vi "Find API Tester Path.vi"(8 "error in":errorcluster, 11 "DQMH Library Ref":refnum<vi>) -> (0 "error out":errorcluster, 3 "API Tester Path":path)   [LabVIEW 2020, in "Dashboard.lvlib"]
uses:
  Dashboard.lvlib
  <vilib>/Utility/error.llb/Error Cluster From Error Code.vi
  <vilib>/ErrorRing/Error Ring.xnode
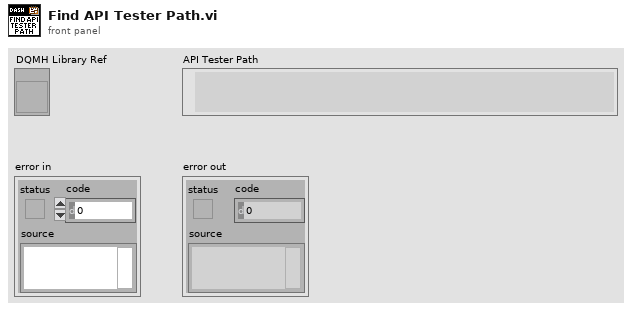
[diagram p1: front panel]
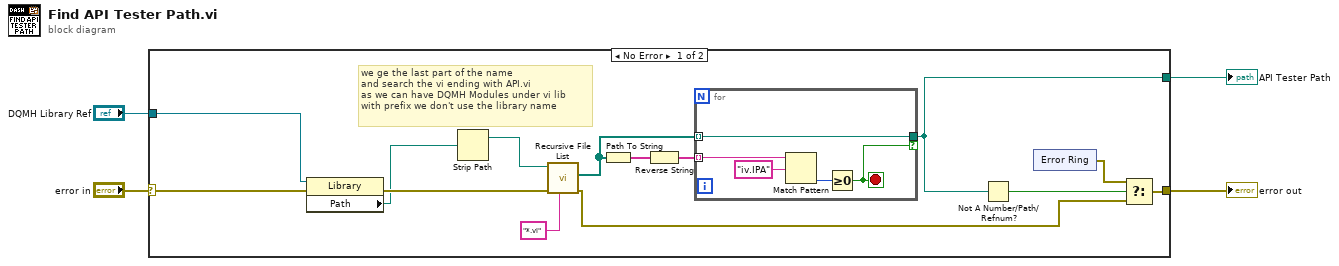
[diagram p0: block diagram]
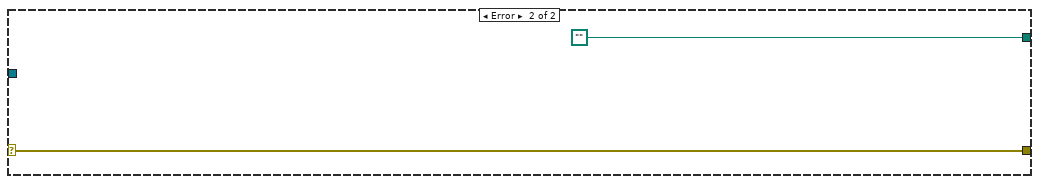
[diagram p2: hidden frame]
diagram:
  n1 = case shown="No Error" "error in" {
    selector: "error in" -> [w14 w30]
    tunnel: [w6 path ""] -> w2
    tunnel: [w16 w30] -> w3
    tunnel: "DQMH Library Ref" -> [w7 _]
    frame No Error {
      # "we ge the last part of the name\nand search the vi ending with API.vi\nas we can have DQMH Modules under vi lib\nwith prefix we don't use the library name"
      n2 = property class="Library"(reference=w7, error in=w14) -> (error out=w15:errorcluster, "Path"=w8:path)  [unwired: 1 out]
      n3 = Strip Path(path=w8) -> (stripped path=w9:path)  [unwired: 1 out]
      n4 = call <vilib>:"Recursive File List.vi"("pattern"="*.vi", "error in (no error)"=w15, "Folder Path"=w9) -> ("error out"=w17:errorcluster, "All Files in Dir"=w10:path[])  [unwired: 4 in, 3 out]
      n5 = Path To String(path=w10) -> (string=w12:string[])
      n6 = Reverse String(1:w12) -> (0:w11:string[])
      n7 = for {
        tunnel: w11 -> [w26] mode=indexing
        tunnel: w10 -> [w28] mode=indexing
        tunnel: [w28] -> w6 if=w24
        stop <- w24 stop-if-true
        n8 = Match Pattern(string=w26, regular expression="iv.IPA") -> (offset past match=w25:i32)  [unwired: 1 in, 3 out]
        n9 = Greater Or Equal To 0?(x=w25) -> (x >= 0?=w24:bool)
      }
      n10 = Not A Number/Path/Refnum?(number/path/refnum=w6) -> (NaN/Path/Refnum?=w5:bool)
      n11 = xnode "Error Ring"() -> ("error out"=w18:errorcluster)
      n12 = Select(t=w18, s=w5, f=w17) -> (s? t:f=w16:errorcluster)
    }
    frame Error {
    }
  }
  "API Tester Path" <- w2
  "error out" <- w3
